vi "3asortingevennum.vi"() -> ()   [LabVIEW 2013]
panel:
  out "Array":dbl[](array[numeric])
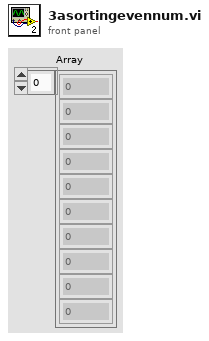
[diagram p1: front panel]
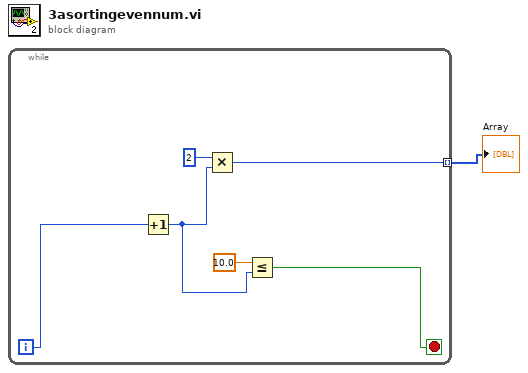
[diagram p0: block diagram]
diagram:
  n1 = while {
    tunnel: [w2] -> w1 mode=indexing
    i -> [w7]
    stop <- w6 stop-if-true
    n2 = Increment(x=w7) -> (x+1=w3:i32)
    n3 = Multiply(x=2, y=w3) -> (x*y=w2:i32)
    n4 = Less Or Equal?(x=10.0, y=w3) -> (x <= y?=w6:bool)
  }
  "Array" <- w1
